vi "left_side_centralize.vi"(0 "samples":i32, 1 "step(mm)":i32, 2 "inner_b_ir":dbl, 3 "inner_f_ir":dbl) -> ()   [LabVIEW 2017]
uses:
  <vilib>/myRIO/Instrument Drivers/Onboard IO/AI/typedefs/AI Reference.ctl
  <vilib>/myRIO/Common/Instrument Driver Framework/Utilities/typedefs/myRIO Generic Hardware Reference.ctl
  <vilib>/myRIO/Common/Instrument Driver Framework/Utilities/typedefs/Hardware Version Enum.ctl
  <vilib>/myRIO/Common/Instrument Driver Framework/Utilities/typedefs/myRIO v1.0 Reference.ctl
  <vilib>/myRIO/Common/Instrument Driver Framework/Utilities/typedefs/Generic FPGA Reference.ctl
  <vilib>/myRIO/Common/Instrument Driver Framework/myRIO v1.0/AI/typedefs/AI Channels List.ctl
  <vilib>/myRIO/Common/Instrument Driver Framework/myRIO v1.0/AI/typedefs/AI Channels Enum.ctl
  <vilib>/myRIO/Common/Instrument Driver Framework/Utilities/typedefs/Analog Scaling Constants List.ctl
  <vilib>/myRIO/Common/Instrument Driver Framework/Utilities/typedefs/Analog Scaling Constants.ctl
  <vilib>/userdefined/High Color/nirio_resource_hc.ctl
  <vilib>/myRIO/Common/Instrument Driver Framework/Utilities/vis/Is FPGA Ref Available.vi
  <vilib>/myRIO/Common/Instrument Driver Framework/myRIO v1.0/AI/vis/myRIO v1.1 Open AI.vi
  <vilib>/myRIO/Instrument Drivers/Onboard IO/AI/vis/Read.vi
  <vilib>/Analysis/baseanly.llb/Mean (DBL).vi
  <vilib>/myRIO/Common/Instrument Driver Framework/Utilities/vis/Validate Channels.vi
  <vilib>/myRIO/Common/Instrument Driver Framework/myRIO v1.0/AI/vis/myRIO v1.0 Reserve AI.vi
  <vilib>/myRIO/Common/Instrument Driver Framework/myRIO v1.0/AI/vis/myRIO v1.0 Build MUX Configuration AI.vi
  <vilib>/myRIO/Common/Instrument Driver Framework/myRIO v1.0/Resource Manager/vis/myRIO v1.0 Reserve Channel List.vi
  <vilib>/myRIO/Common/Instrument Driver Framework/myRIO v1.0/Resource Manager/vis/myRIO v1.0 Reserve Channel.vi
  <vilib>/myRIO/Common/Instrument Driver Framework/myRIO v1.0/Resource Manager/vis/myRIO v1.0 Unreserve Channel.vi
  <vilib>/myRIO/Common/Instrument Driver Framework/myRIO v1.0/Resource Manager/vis/myRIO v1.0 Build Mutex Name.vi
  <vilib>/Utility/VariantDataType/GetNumericInfo.vi
  <vilib>/Utility/error.llb/Error Cluster From Error Code.vi
  <vilib>/myRIO/Common/Instrument Driver Framework/myRIO v1.0/myRIO v1.1 Open.vi
  <vilib>/myRIO/Common/Instrument Driver Framework/myRIO v1.0/AI/vis/myRIO v1.0 Get Scaling Constants AI.vi
  <vilib>/myRIO/Common/Instrument Driver Framework/Utilities/vis/IO Manager.vi
  <vilib>/myRIO/Common/Instrument Driver Framework/Utilities/vis/Configuration Manager.vi
  <vilib>/myRIO/Common/Instrument Driver Framework/myRIO v1.0/myRIO v1.0 Close.vi
  <vilib>/myRIO/Common/Instrument Driver Framework/myRIO v1.0/AI/vis/myRIO v1.0 Read AI.vi
  GlobalVar.vi
  <vilib>/myRIO/Express VI/Onboard IO/AI/AI Express VI.xnode
  <vilib>/myRIO/Instrument Drivers/Onboard IO/AI/vis/myRIO AI Open.xnode
  <vilib>/Analysis/NI_AALBase.lvlib
  <vilib>/myRIO/Instrument Drivers/Onboard IO/AI/AI.lvlib
panel:
  out "pre_r":i32
  out "pre_l":i32
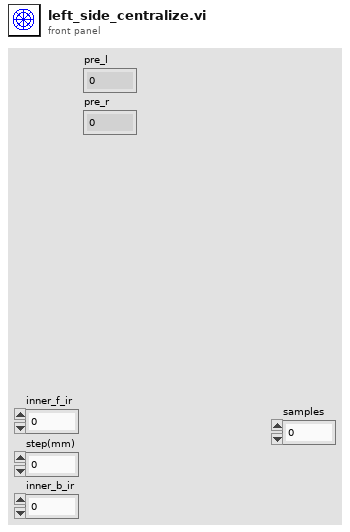
[diagram p1: front panel]
types:
  T1 = typedef "AI.lvlib/AI Reference.ctl" = cluster{"myRIO Reference":T2, "AI Channels List":T6, "AI Scaling Constants List":T8}
  T2 = typedef "myRIO Generic Hardware Reference.ctl" = cluster{"myRIO Model":T3, "myRIO Hardware Reference":T4}
  T3 = typedef "Hardware Version Enum.ctl" = enum16{"Unknown", "myRIO-1900", "myRIO-1950", "roboRIO", "NI ELVIS RIO CM"}
  T4 = typedef "myRIO v1.0 Reference.ctl" = cluster{"Generic FPGA Reference":T5, "Allow multiple opens":bool}
  T5 = typedef "Generic FPGA Reference.ctl" = refnum<k20>
  T6 = typedef "AI Channels List.ctl" = T7[]
  T7 = typedef "AI Channels Enum.ctl" = enum16{"Not Connected", "AudioIn/Left", "AudioIn/Right", "C/AI0", "C/AI1", "A/AI0", "A/AI1", "A/AI2", "A/AI3", "B/AI0", "B/AI1", "B/AI2", "B/AI3", "AI/AI0", "AI/AI1", "AI/AI2", "AI/AI3"}
  T8 = typedef "Analog Scaling Constants List.ctl" = T9[]
  T9 = typedef "Analog Scaling Constants.ctl" = cluster{"LSB Weight (Volts)":dbl, "Offset (Volts)":dbl, "Signed?":bool}
  T10 = typedef "nirio_resource_hc.ctl" = tag
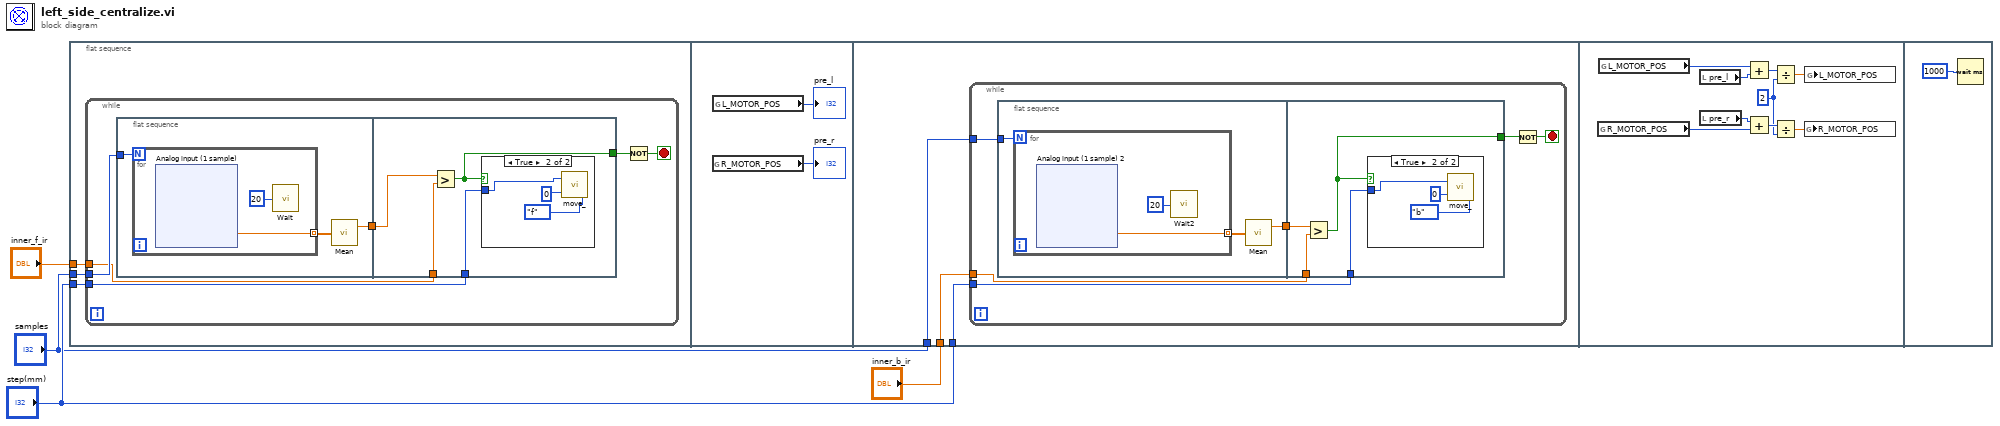
[diagram p0: block diagram]
diagram:
  n1 = flat-sequence {
    tunnel: "samples" -> [w7]
    tunnel: "inner_f_ir" -> [w6]
    tunnel: "step(mm)" -> [w5]
    tunnel: "step(mm)" -> [w67]
    tunnel: "inner_b_ir" -> [w66]
    tunnel: "samples" -> [w65]
    frame #0 {
      n2 = while {
        tunnel: w7 -> [w13]
        tunnel: w6 -> [w11]
        tunnel: w5 -> [w10]
        stop <- w9 stop-if-true
        n3 = flat-sequence {
          tunnel: w13 -> [w15]
          tunnel: [w14] -> w12
          tunnel: w12 -> [w59]
          tunnel: w11 -> [w58]
          tunnel: w10 -> [w57]
          tunnel: [w56] -> w8
          frame #0 {
            n4 = for {
              N: w15 -> [_]
              tunnel: [w18] -> w16 mode=indexing
              n5 = xnode "Analog input (1 sample)"() -> ("lf (B/AI2 (Pin 7))"=w18:dbl)  [unwired: 1 in, 1 out]
              n6 = call "Wait"("Count(uSec)"=u32 20) -> ()  [unwired: 1 out]
            }
            n7 = call-poly <vilib>:"Mean.vi"("X"=w16) -> ("mean"=w14:dbl)  [unwired: 1 out]
          }
          frame #1 {
            n8 = Greater?(x=w59, y=w58) -> (0:w56:bool)
            n9 = case shown="True" w56 {
              tunnel: w57 -> [_ w62]
              frame False {
              }
              frame True {
                n10 = call "move_.vi"("Enum"=enum16{"hold", "f", "b"}."f", "delay"=u32 0, "D"=w62) -> ()  [unwired: 1 in]
              }
            }
          }
        }
        n11 = Not(x=w8) -> (.not. x?=w9:bool)
      }
    }
    frame #1 {
      n12 = global read "GlobalVar.vi" "R_MOTOR_POS"() -> (→"pre_r":i32)
      n13 = global read "GlobalVar.vi" "L_MOTOR_POS"() -> (→"pre_l":i32)
    }
    frame #2 {
      n14 = while {
        tunnel: w67 -> [w72]
        tunnel: w66 -> [w69]
        tunnel: w65 -> [w68]
        stop <- w71 stop-if-true
        n15 = flat-sequence {
          tunnel: [w76] -> w73
          tunnel: w68 -> [w74]
          tunnel: w73 -> [w119]
          tunnel: w72 -> [w118]
          tunnel: [w117] -> w70
          tunnel: w69 -> [w116]
          frame #0 {
            n16 = for {
              N: w74 -> [_]
              tunnel: [w78] -> w75 mode=indexing
              n17 = xnode "Analog input (1 sample) 2"() -> ("lb (B/AI3 (Pin 9))"=w78:dbl)  [unwired: 1 in, 1 out]
              n18 = call "Wait2"("Count(uSec)"=u32 20) -> ()  [unwired: 1 out]
            }
            n19 = call-poly <vilib>:"Mean.vi"("X"=w75) -> ("mean"=w76:dbl)  [unwired: 1 out]
          }
          frame #1 {
            n20 = Greater?(x=w119, y=w116) -> (0:w117:bool)
            n21 = case shown="True" w117 {
              tunnel: w118 -> [_ w122]
              frame False {
              }
              frame True {
                n22 = call "move_.vi"("Enum"=enum16{"hold", "f", "b"}."b", "delay"=u32 0, "D"=w122) -> ()  [unwired: 1 in]
              }
            }
          }
        }
        n23 = Not(x=w70) -> (.not. x?=w71:bool)
      }
    }
    frame #3 {
      w125 = 2 ("y")
      n24 = global read "GlobalVar.vi" "R_MOTOR_POS"() -> (w130:i32)
      n25 = global read "GlobalVar.vi" "L_MOTOR_POS"() -> (w131:i32)
      n26 = local read "pre_l"() -> (w129:i32)
      n27 = local read "pre_r"() -> (w128:i32)
      n28 = Add(x=w131, y=w129) -> (x+y=w127:i32)
      n29 = Add(x=w128, y=w130) -> (x+y=w126:i32)
      n30 = Divide(x=w127, y=w125) -> (x/y=w123:dbl)
      n31 = Divide(x=w126, y=w125) -> (x/y=w124:dbl)
      n32 = global write "GlobalVar.vi" "R_MOTOR_POS"(w124) -> ()
      n33 = global write "GlobalVar.vi" "L_MOTOR_POS"(w123) -> ()
    }
    frame #4 {
      n34 = Wait (ms)(milliseconds to wait=u32 1000) -> ()  [unwired: 1 out]
    }
  }
